vi "ReadAlgoParametersJSON_General.vi"(8 "error in":errorcluster, 10 "Algo Override\nJSON Variant in":variant, 11 "Read Edit Tolerance \nOverride JSON":path=path "C:/Users/raakeshs/Desktop/GTRON/JSONs/DeafultJSON_Final.json") -> (0 "error out":errorcluster, 2 "Variant":variant, 3 "ZenGage v3.0 UI.lvclass:Algo(Override)_CoeffficientsIncluded":T1)   [LabVIEW 2019, in "ZenGage v3.0 UI.lvclass"]
uses:
  ZenGage v3.0 UI.lvclass
  Type Definitions/JSON Read/Algo(Override)_CoeffficientsIncluded.ctl
panel:
  out "VCluster\n out":variant
  out "Error Message":string
types:
  T1 = typedef "ZenGage v3.0 UI.lvclass/Algo(Override)_CoeffficientsIncluded.ctl" = cluster{"AlgoParameters":cluster{"PartsList":cluster{"Name":string, "Measurements":cluster{"RackID":dbl, "MeasurementId":dbl, "Name":string, "AlgoName":string, "MeasurementEnable":bool, "UserCalibCoefficients":cluster{"UserCorrectionLinearityCoeff":dbl, "UserCorrectionBiasCoeff":dbl}, "SpecValues":cluster{"LCL":dbl, "UCL":dbl, "LSL":dbl, "USL":dbl, "NominalValue":dbl}}[]}[]}}
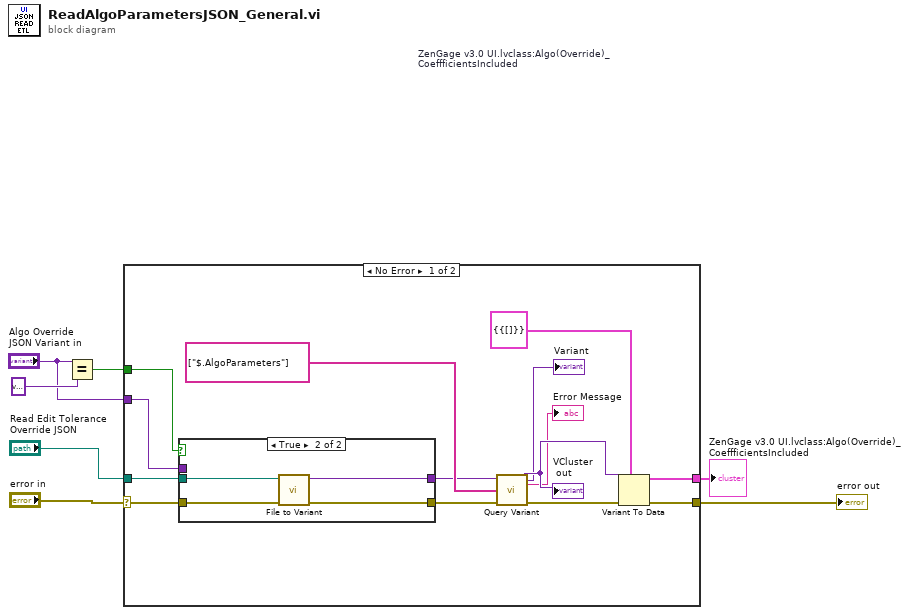
[diagram p0: block diagram]
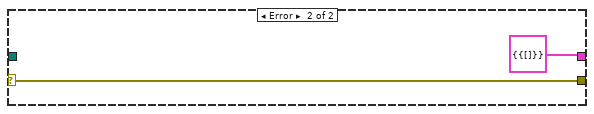
[diagram p3: hidden frame]
diagram:
  n1 = Equal?(x="Algo Override\nJSON Variant in", y=variant) -> (x = y?=w1:bool)
  n2 = case shown="No Error" "error in" {
    selector: "error in" -> [w16 w28]
    tunnel: [w18 w28] -> w7
    tunnel: "Read Edit Tolerance \nOverride JSON" -> [w15 _]
    tunnel: "Algo Override\nJSON Variant in" -> [w11 _]
    tunnel: w1 -> [w10 _]
    tunnel: [w8 T1 {"AlgoParameters"={"PartsList"=[]}} ("ZenGage v3.0 UI.lvclass:Algo(Override)_CoeffficientsIncluded")] -> w2
    frame No Error {
      w9 = T1 {"AlgoParameters"={"PartsList"=[]}}  # ZenGage v3.0 UI.lvclass:Algo(Override)_CoeffficientsIncluded
      n3 = case shown="True" w10 {
        tunnel: w16 -> [w22 w26]
        tunnel: w15 -> [_ w25]
        tunnel: [w22 w23] -> w13
        tunnel: [w21 w24] -> w12
        tunnel: w11 -> [w21 _]
        frame False {
        }
        frame True {
          n4 = call <vilib>:"File to Variant.vi"("JSON FilePath"=w25, "error in (no error)"=w26) -> ("JSON Variant"=w24:variant, "error out"=w23:errorcluster)  [unwired: 6 in, 1 out]
        }
      }
      "Variant" <- w12
      n5 = call <vilib>:"Query Variant.vi"("VCluster in"=w12, "pathList"=string[] ["$.AlgoParameters"], "error IO"=w13) -> ("VCluster\n out"=w20:variant, "Error Message"=→"Error Message":string, "error out"=w19:errorcluster)  [unwired: 9 in, 1 out]
      "VCluster\n out" <- w20
      n6 = Variant To Data(error in=w19, type=w9, Variant=w20) -> (data=w8:T1, error out=w18:errorcluster)
    }
    frame Error {
    }
  }
  "error out" <- w7
  "ZenGage v3.0 UI.lvclass:Algo(Override)_CoeffficientsIncluded" <- w2
